vi "Bin Data.vi"(9 "Bins around center":dbl, 10 "Bin Width (pixels)":dbl=1.0 min=1.0 max=1024.0 step=1.0, 11 "Pixel data":i32[](array[numeric])) -> (8 "Array of Wavelengths":dbl[](array[numeric]))   [LabVIEW 2017, in "Synapse CCD.lvclass"]
uses:
  Synapse CCD.lvclass
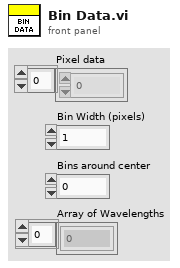
[diagram p1: front panel]
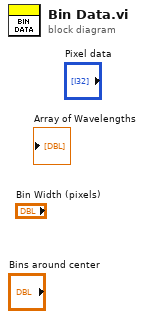
[diagram p0: block diagram]
diagram:
